vi "CSP_Weight_Calculator.vi"(8 "X4_Down movement":path, 9 "X3_Up movement":path, 10 "X2_Left movement":path, 11 "X1_Right movement":path) -> (0 "WL4":T1, 1 "WL3":T1, 2 "WL2":T1, 3 "WL1":T1)   [LabVIEW 2014]
uses:
  <vilib>/Analysis/Matrix/Datatypes/RealMatrix.ctl
  <vilib>/Analysis/baseanly.llb/Real A x B.vi
  <vilib>/Analysis/baseanly.llb/Complex A x B.vi
  <vilib>/Utility/file.llb/Read From Spreadsheet File (DBL).vi
  <vilib>/Analysis/Matrix/Numeric/Add/Add - RM,RM.vi
  <vilib>/Analysis/7linalg.llb/Real Eigenvalues and Vectors.vi
  <vilib>/Analysis/Matrix/Numeric/Complex/Complex To Cartesian - CM.vi
  <vilib>/Analysis/NI_AALBase.lvlib
  <vilib>/Analysis/Matrix/NI_Matrix.lvlib
  <vilib>/Analysis/NI_AALPro.lvlib
panel:
  out "P":T1
  out "C4":T1
  out "C3":T1
  out "C2":T1
  out "C1":T1
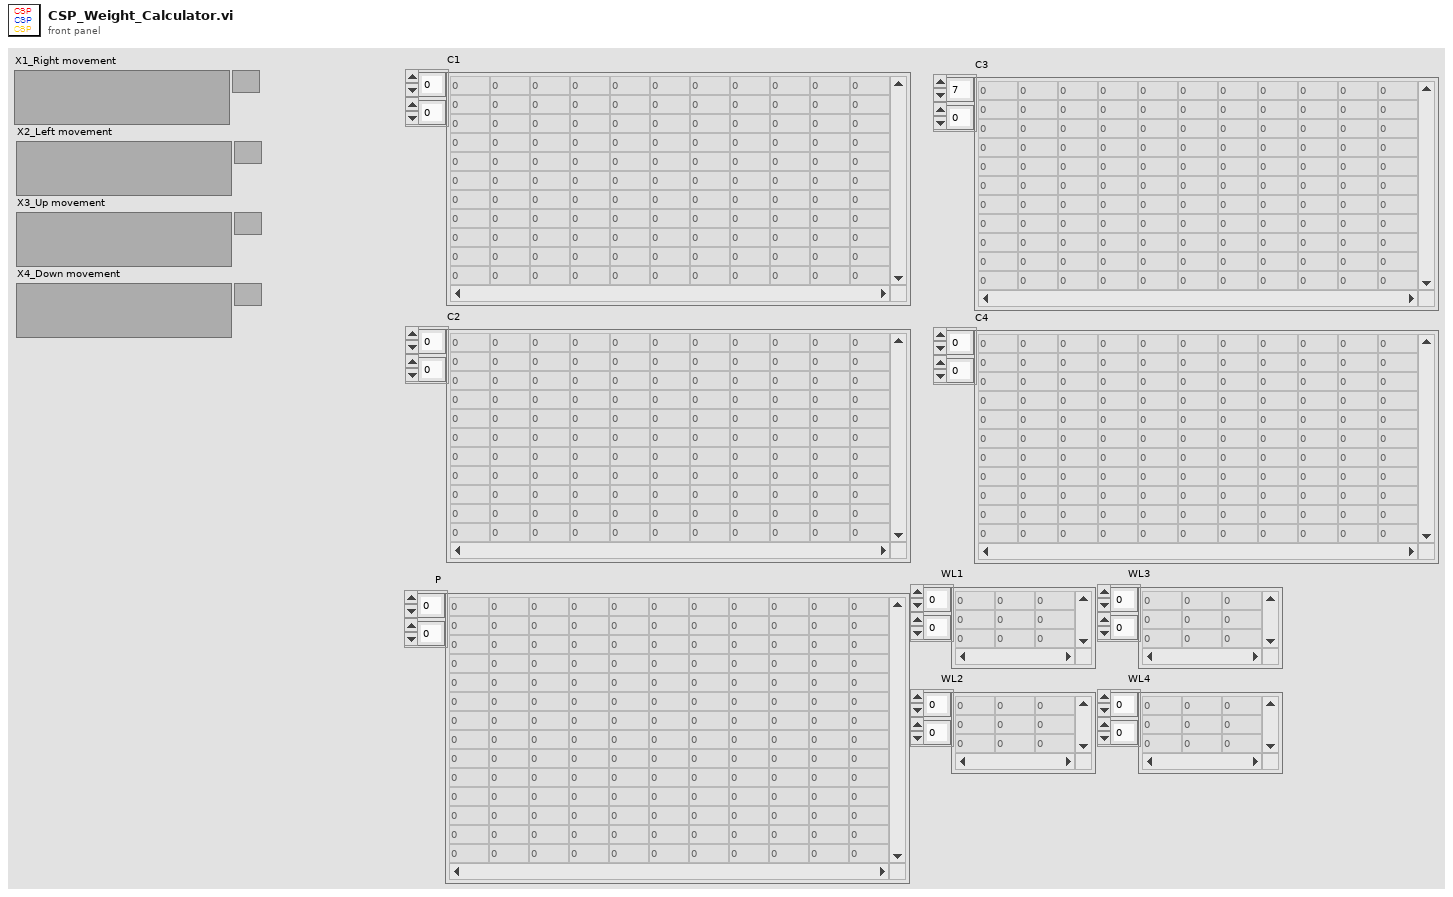
[diagram p1: front panel]
types:
  T1 = typedef "NI_Matrix.lvlib/RealMatrix.ctl" = dbl[][]
  T2 = typedef "NI_Matrix.lvlib/ComplexMatrix.ctl" = cdb[][]
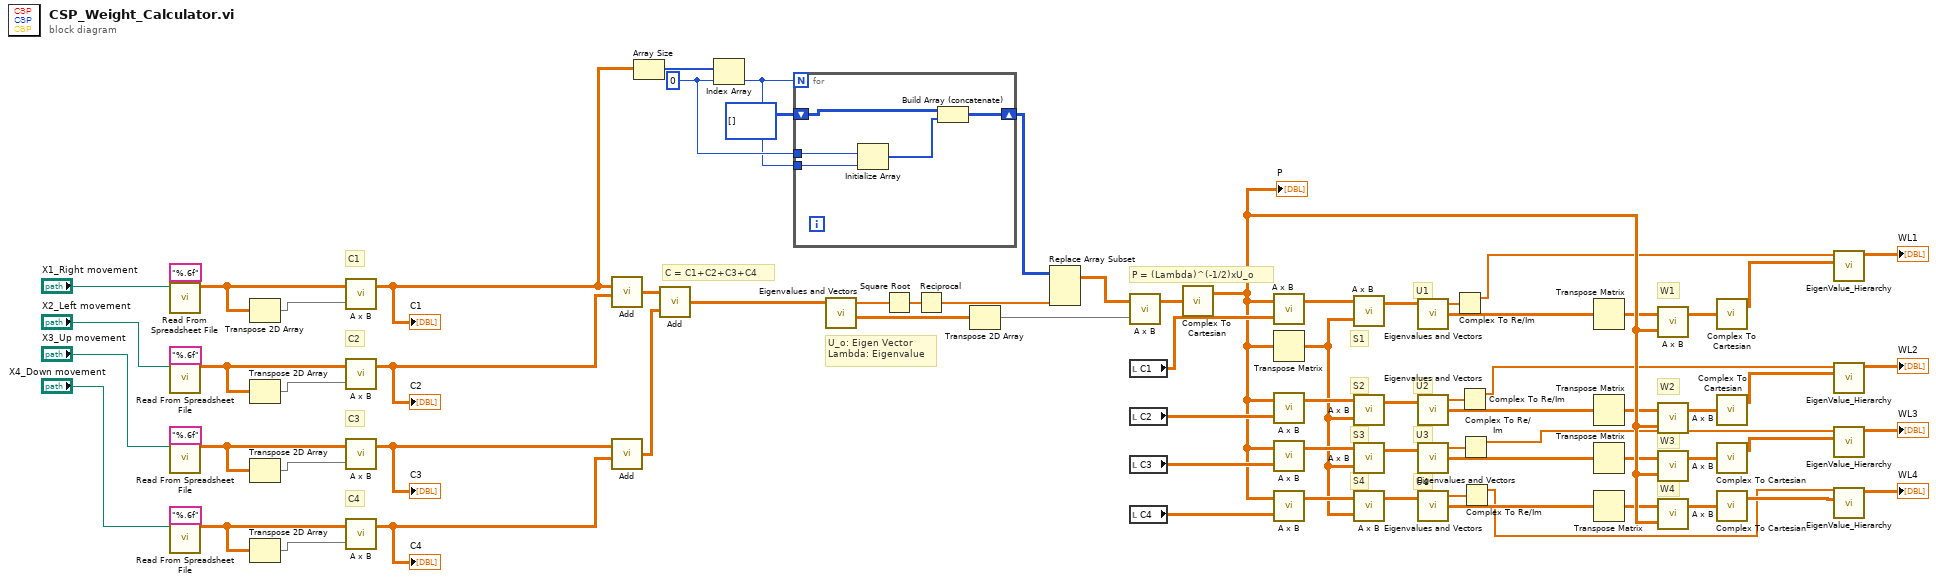
[diagram p0: block diagram]
diagram:
  w52 = 0 ("index")
  # "W4"
  # "W3"
  # "W2"
  # "W1"
  # "U4"
  # "U3"
  # "U2"
  # "U1"
  # "S4"
  # "S3"
  # "S2"
  # "S1"
  # "P = (Lambda)^(-1/2)xU_o"
  # "U_o: Eigen Vector\nLambda: Eigenvalue"
  # "C = C1+C2+C3+C4"
  # "C4"
  # "C3"
  # "C2"
  # "C1"
  n1 = call-poly <vilib>:"Read From Spreadsheet File.vi"("format (%.3f)"="%.6f", "file path (dialog if empty)"="X1_Right movement") -> ("all rows"=w69:dbl[][])  [unwired: 5 in, 4 out]
  n2 = call-poly <vilib>:"Read From Spreadsheet File.vi"("format (%.3f)"="%.6f", "file path (dialog if empty)"="X2_Left movement") -> ("all rows"=w66:dbl[][])  [unwired: 5 in, 4 out]
  n3 = call-poly <vilib>:"Read From Spreadsheet File.vi"("format (%.3f)"="%.6f", "file path (dialog if empty)"="X3_Up movement") -> ("all rows"=w65:dbl[][])  [unwired: 5 in, 4 out]
  n4 = call-poly <vilib>:"Read From Spreadsheet File.vi"("format (%.3f)"="%.6f", "file path (dialog if empty)"="X4_Down movement") -> ("all rows"=w63:dbl[][])  [unwired: 5 in, 4 out]
  n5 = Transpose 2D Array(2D array=w69) -> (transposed array=w68:dbl[][])
  n6 = Transpose 2D Array(2D array=w66) -> (transposed array=w67:dbl[][])
  n7 = Transpose 2D Array(2D array=w65) -> (transposed array=w64:dbl[][])
  n8 = Transpose 2D Array(2D array=w63) -> (transposed array=w62:dbl[][])
  n9 = call-poly <vilib>:"A x B.vi"("B"=w68, "A"=w69) -> ("A x B"=w54:T1)  [unwired: 1 out]
  "C1" <- w54
  n10 = call-poly <vilib>:"A x B.vi"("B"=w67, "A"=w66) -> ("A x B"=w46:T1)  [unwired: 1 out]
  "C2" <- w46
  n11 = call-poly <vilib>:"A x B.vi"("B"=w64, "A"=w65) -> ("A x B"=w45:T1)  [unwired: 1 out]
  "C3" <- w45
  n12 = call-poly <vilib>:"A x B.vi"("B"=w62, "A"=w63) -> ("A x B"=w44:T1)  [unwired: 1 out]
  "C4" <- w44
  n13 = call-poly <vilib>:"Add.vi"("Real Matrix B"=w46, "Real Matrix A"=w54) -> ("A + B"=w61:T1)
  n14 = call-poly <vilib>:"Add.vi"("Real Matrix B"=w44, "Real Matrix A"=w45) -> ("A + B"=w60:T1)
  n15 = Array Size(array=w54) -> (size(s)=w53:i32[])
  n16 = call-poly <vilib>:"Add.vi"("Real Matrix B"=w60, "Real Matrix A"=w61) -> ("A + B"=w59:T1)
  n17 = Index Array(array=w53, index=w52) -> (element=w51:i32)
  n18 = for {
    N: w51 -> [_]
    tunnel: w52 -> [w82]
    tunnel: w51 -> [w81]
    shift-right: [w79] -> w49
    shift-left: i32[][] [] -> [w78]
    n19 = Initialize Array(w82, w81) -> (w80:i32[])
    n20 = Build Array (concatenate)(w78, w80) -> (w79:i32[][])
  }
  n21 = call-poly <vilib>:"Eigenvalues and Vectors.vi"("Input Matrix"=w59) -> ("Eigenvectors"=w56:T2, "Eigenvalues"=w58:cdb[])  [unwired: 2 in, 1 out]
  n22 = Square Root(x=w58) -> (sqrt(x)=w57:cdb[])
  n23 = Reciprocal(x=w57) -> (1/x=w55:cdb[])
  n24 = Transpose 2D Array(2D array=w56) -> (transposed array=w47:T2)
  n25 = Replace Array Subset(array=w49, new element=w55) -> (w48:T2)  [unwired: 2 in]
  n26 = call-poly <vilib>:"A x B.vi"("B"=w47, "A"=w48) -> ("A x B"=w30:T2)  [unwired: 1 out]
  n27 = local read "C1"() -> (w43:T1)
  n28 = local read "C2"() -> (w41:T1)
  n29 = local read "C3"() -> (w40:T1)
  n30 = local read "C4"() -> (w39:T1)
  n31 = call-poly <vilib>:"Complex To Cartesian.vi"("Complex Matrix R + Ii"=w30) -> ("Real Matrix R"=w25:T1)  [unwired: 1 out]
  "P" <- w25
  n32 = call-poly <vilib>:"A x B.vi"("B"=w43, "A"=w25) -> ("A x B"=w42:T1)  [unwired: 1 out]
  n33 = Transpose Matrix(1:w25) -> (0:w35:T1)
  n34 = call-poly <vilib>:"A x B.vi"("B"=w41, "A"=w25) -> ("A x B"=w38:T1)  [unwired: 1 out]
  n35 = call-poly <vilib>:"A x B.vi"("B"=w40, "A"=w25) -> ("A x B"=w37:T1)  [unwired: 1 out]
  n36 = call-poly <vilib>:"A x B.vi"("B"=w39, "A"=w25) -> ("A x B"=w36:T1)  [unwired: 1 out]
  n37 = call-poly <vilib>:"A x B.vi"("B"=w35, "A"=w42) -> ("A x B"=w34:T1)  [unwired: 1 out]
  n38 = call-poly <vilib>:"A x B.vi"("B"=w35, "A"=w38) -> ("A x B"=w33:T1)  [unwired: 1 out]
  n39 = call-poly <vilib>:"A x B.vi"("B"=w35, "A"=w37) -> ("A x B"=w32:T1)  [unwired: 1 out]
  n40 = call-poly <vilib>:"A x B.vi"("B"=w35, "A"=w36) -> ("A x B"=w31:T1)  [unwired: 1 out]
  n41 = call-poly <vilib>:"Eigenvalues and Vectors.vi"("Input Matrix"=w34) -> ("Eigenvectors"=w29:T2, "Eigenvalues"=w16:cdb[])  [unwired: 2 in, 1 out]
  n42 = call-poly <vilib>:"Eigenvalues and Vectors.vi"("Input Matrix"=w33) -> ("Eigenvectors"=w28:T2, "Eigenvalues"=w15:cdb[])  [unwired: 2 in, 1 out]
  n43 = call-poly <vilib>:"Eigenvalues and Vectors.vi"("Input Matrix"=w32) -> ("Eigenvectors"=w27:T2, "Eigenvalues"=w14:cdb[])  [unwired: 2 in, 1 out]
  n44 = call-poly <vilib>:"Eigenvalues and Vectors.vi"("Input Matrix"=w31) -> ("Eigenvectors"=w26:T2, "Eigenvalues"=w13:cdb[])  [unwired: 2 in, 1 out]
  n45 = Complex To Re/Im ("Complex To Cartesian.vi")(x + iy=w16) -> (x=w11:dbl[])  [unwired: 1 out]
  n46 = Complex To Re/Im ("Complex To Cartesian.vi")(x + iy=w15) -> (x=w9:dbl[])  [unwired: 1 out]
  n47 = Complex To Re/Im ("Complex To Cartesian.vi")(x + iy=w14) -> (x=w7:dbl[])  [unwired: 1 out]
  n48 = Complex To Re/Im ("Complex To Cartesian.vi")(x + iy=w13) -> (x=w5:dbl[])  [unwired: 1 out]
  n49 = Transpose Matrix(1:w29) -> (0:w24:T2)
  n50 = Transpose Matrix(1:w28) -> (0:w23:T2)
  n51 = Transpose Matrix(1:w27) -> (0:w22:T2)
  n52 = Transpose Matrix(1:w26) -> (0:w21:T2)
  n53 = call-poly <vilib>:"A x B.vi"("B"=w25, "A"=w24) -> ("A x B"=w20:T2)  [unwired: 1 out]
  n54 = call-poly <vilib>:"A x B.vi"("B"=w25, "A"=w23) -> ("A x B"=w19:T2)  [unwired: 1 out]
  n55 = call-poly <vilib>:"A x B.vi"("B"=w25, "A"=w22) -> ("A x B"=w18:T2)  [unwired: 1 out]
  n56 = call-poly <vilib>:"A x B.vi"("B"=w25, "A"=w21) -> ("A x B"=w17:T2)  [unwired: 1 out]
  n57 = call-poly <vilib>:"Complex To Cartesian.vi"("Complex Matrix R + Ii"=w20) -> ("Real Matrix R"=w12:T1)  [unwired: 1 out]
  n58 = call-poly <vilib>:"Complex To Cartesian.vi"("Complex Matrix R + Ii"=w19) -> ("Real Matrix R"=w10:T1)  [unwired: 1 out]
  n59 = call-poly <vilib>:"Complex To Cartesian.vi"("Complex Matrix R + Ii"=w18) -> ("Real Matrix R"=w8:T1)  [unwired: 1 out]
  n60 = call-poly <vilib>:"Complex To Cartesian.vi"("Complex Matrix R + Ii"=w17) -> ("Real Matrix R"=w6:T1)  [unwired: 1 out]
  n61 = call "EigenValue_Hierarchy.vi"("Weight Array (Wx)"=w12, "EigenValues"=w11) -> ("WL"=→"WL1":dbl[][])  [unwired: 9 in]
  n62 = call "EigenValue_Hierarchy.vi"("Weight Array (Wx)"=w10, "EigenValues"=w9) -> ("WL"=→"WL2":dbl[][])  [unwired: 9 in]
  n63 = call "EigenValue_Hierarchy.vi"("Weight Array (Wx)"=w8, "EigenValues"=w7) -> ("WL"=→"WL3":dbl[][])  [unwired: 9 in]
  n64 = call "EigenValue_Hierarchy.vi"("Weight Array (Wx)"=w6, "EigenValues"=w5) -> ("WL"=→"WL4":dbl[][])  [unwired: 9 in]
